vi "dds writer config to reader.vi"(11 "writer configuration":T1) -> (3 "reader configuration":T2)   [LabVIEW 2020, in "DDS configuration.lvclass"]
uses:
  dds configuration.lvclass
  <vilib>/RTI DDS Toolkit/Types/RTI DDS Advanced Reader Configuration.ctl
  <vilib>/RTI DDS Toolkit/Types/RTI DDS Advanced Writer Configuration.ctl
  <vilib>/RTI DDS Toolkit/Library/LVDDS_library.lvlib
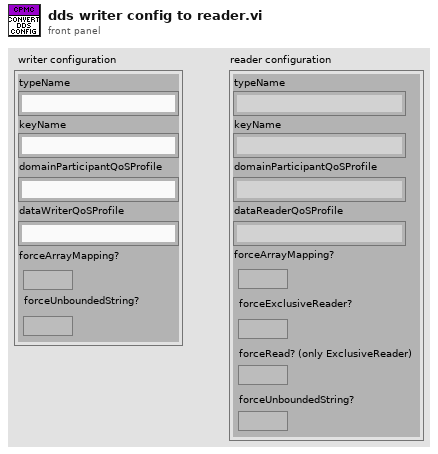
[diagram p1: front panel]
types:
  T1 = typedef "LVDDS_library.lvlib/RTI DDS Advanced Writer Configuration.ctl" = cluster{"typeName":string, "keyName":string, "domainParticipantQoSProfile":string, "dataWriterQoSProfile":string, "forceArrayMapping?":bool, "forceUnboundedString?":bool}
  T2 = typedef "LVDDS_library.lvlib/RTI DDS Advanced Reader Configuration.ctl" = cluster{"typeName":string, "keyName":string, "domainParticipantQoSProfile":string, "dataReaderQoSProfile":string, "forceArrayMapping?":bool, "forceExclusiveReader?":bool, "forceRead? (only ExclusiveReader)":bool, "forceUnboundedString?":bool}
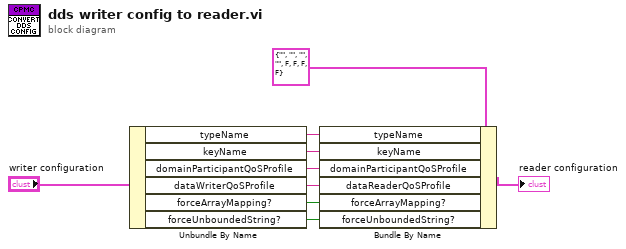
[diagram p0: block diagram]
diagram:
  n1 = Unbundle By Name("writer configuration") -> ("typeName"=w9:string, "keyName"=w8:string, "domainParticipantQoSProfile"=w7:string, "dataWriterQoSProfile"=w6:string, "forceArrayMapping?"=w5:bool, "forceUnboundedString?"=w4:bool)
  n2 = Bundle By Name(cluster=T2 {"typeName"="", "keyName"="", "domainParticipantQoSProfile"="", "dataReaderQoSProfile"="", "forceArrayMapping?"=FALSE, "forceExclusiveReader?"=FALSE, "forceRead? (only ExclusiveReader)"=FALSE, "forceUnboundedString?"=FALSE} ("reader configuration"), "typeName"=w9, "keyName"=w8, "domainParticipantQoSProfile"=w7, "dataReaderQoSProfile"=w6, "forceArrayMapping?"=w5, "forceUnboundedString?"=w4) -> (→"reader configuration":T2)
